vi "Convert_Algo_Info.vi"(0 "ERD Data Out 1":T1[](array[typedef]) {"ERD Number" format="%.0x"}, 5 "ERD Data Out 2":T1[](array[typedef]) {"ERD Number" format="%.0x"}, 11 "Error In":errorcluster) -> (4 "Algorithm Data":T2, 15 "Error Out":errorcluster)   [LabVIEW 2014]
uses:
  type defs/Algorithms.ctl
  Utility/Labview GEA2 Toolkit v2.1/type defs/ERD Read Data Out.ctl
  Utility/Labview GEA2 Toolkit v2.1/library/GEA2_Toolkit.lvlib
panel:
  # "Wet Load Size"
  # "Dry Load Size"
  # "OOB"
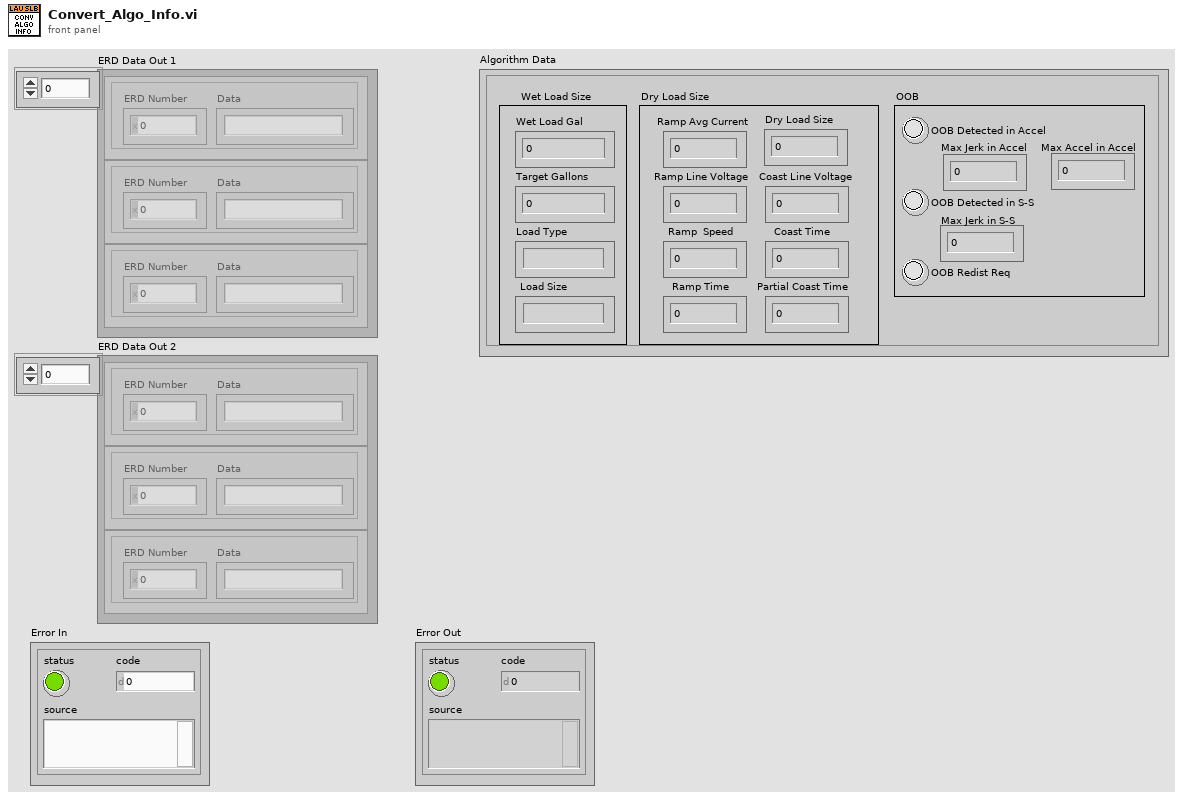
[diagram p1: front panel]
types:
  T1 = typedef "GEA2_Toolkit.lvlib/ERD Read Data Out.ctl" = cluster{"ERD Number":u16, "Data":string}
  T2 = typedef "Algorithms.ctl" = cluster{"Wet Load Gal":dbl, "Target Gallons":dbl, "Load Type":string, "Load Size":string, "Coast Time":u16, "Ramp Time":u16, "Ramp  Speed":u16, "Ramp Avg Current":dbl, "OOB Redist Req":bool, "OOB Detected in S-S":bool, "Max Accel in Accel":i32, "Max Jerk in Accel":i32, "Max Jerk in S-S":i32, "OOB Detected in Accel":bool, "Partial Coast Time":u16, "Dry Load Size":dbl, "Ramp Line Voltage ":dbl, "Coast Line Voltage":dbl}
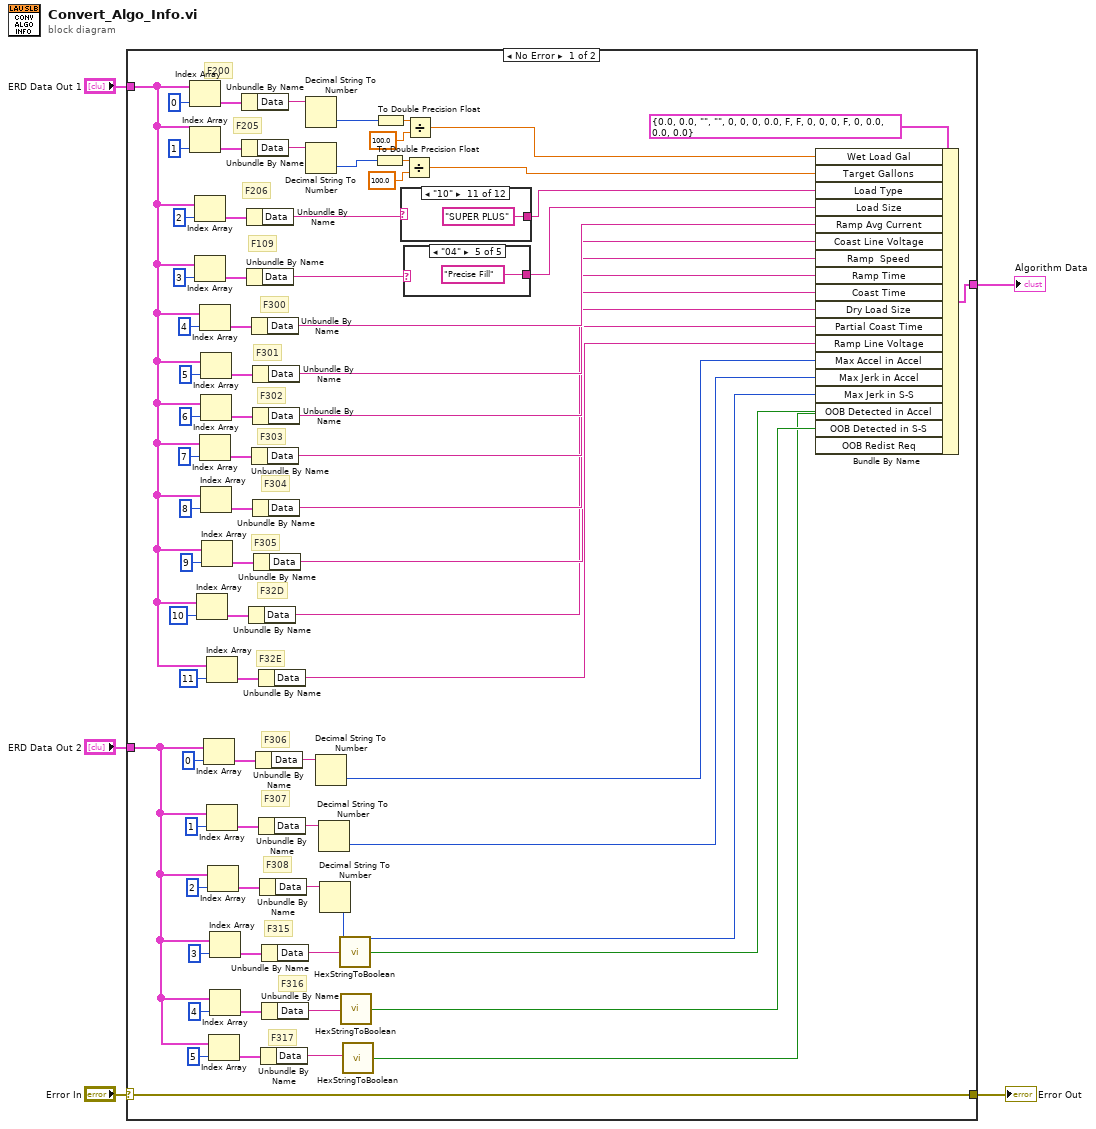
[diagram p0: block diagram]
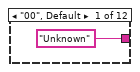
[diagram p2: hidden frame]
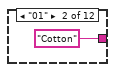
[diagram p3: hidden frame]
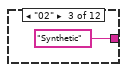
[diagram p4: hidden frame]
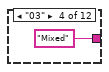
[diagram p5: hidden frame]
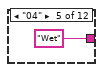
[diagram p6: hidden frame]
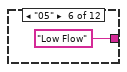
[diagram p7: hidden frame]
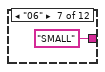
[diagram p8: hidden frame]
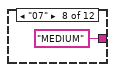
[diagram p9: hidden frame]
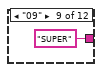
[diagram p10: hidden frame]
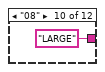
[diagram p11: hidden frame]
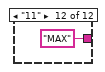
[diagram p12: hidden frame]
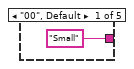
[diagram p13: hidden frame]
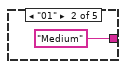
[diagram p14: hidden frame]
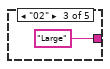
[diagram p15: hidden frame]
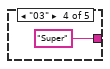
[diagram p16: hidden frame]
diagram:
  n1 = case shown="No Error" "Error In" {
    selector: "Error In" -> [w80 w98]
    tunnel: [w80 w98] -> w4
    tunnel: [w78 _] -> w3
    tunnel: "ERD Data Out 1" -> [w14 _]
    tunnel: "ERD Data Out 2" -> [w25 _]
    frame No Error {
      # "F32E"
      # "F32D"
      # "F317"
      # "F316"
      # "F315"
      # "F308"
      # "F307"
      # "F306"
      # "F305"
      # "F304"
      # "F303"
      # "F302"
      # "F301"
      # "F300"
      # "F109"
      # "F206"
      # "F205"
      # "F200"
      n2 = Index Array(array=w14, index=0) -> (element=w68:T1)
      n3 = Index Array(array=w14, index=1) -> (element=w64:T1)
      n4 = Index Array(array=w14, index=2) -> (element=w60:T1)
      n5 = Index Array(array=w14, index=3) -> (element=w56:T1)
      n6 = Index Array(array=w14, index=10) -> (element=w18:T1)
      n7 = Index Array(array=w14, index=4) -> (element=w58:T1)
      n8 = Index Array(array=w14, index=7) -> (element=w49:T1)
      n9 = Index Array(array=w14, index=5) -> (element=w53:T1)
      n10 = Index Array(array=w14, index=6) -> (element=w52:T1)
      n11 = Index Array(array=w14, index=8) -> (element=w48:T1)
      n12 = Index Array(array=w14, index=9) -> (element=w45:T1)
      n13 = Index Array(array=w25, index=0) -> (element=w44:T1)
      n14 = Index Array(array=w14, index=11) -> (element=w16:T1)
      n15 = Index Array(array=w25, index=1) -> (element=w37:T1)
      n16 = Index Array(array=w25, index=2) -> (element=w36:T1)
      n17 = Index Array(array=w25, index=5) -> (element=w26:T1)
      n18 = Index Array(array=w25, index=3) -> (element=w30:T1)
      n19 = Index Array(array=w25, index=4) -> (element=w29:T1)
      n20 = Unbundle By Name(w68) -> ("Data"=w67:string)
      n21 = Unbundle By Name(w64) -> ("Data"=w65:string)
      n22 = Unbundle By Name(w60) -> ("Data"=w59:string)
      n23 = Unbundle By Name(w56) -> ("Data"=w40:string)
      n24 = Unbundle By Name(w18) -> ("Data"=w7:string)
      n25 = Unbundle By Name(w58) -> ("Data"=w13:string)
      n26 = Unbundle By Name(w49) -> ("Data"=w10:string)
      n27 = Unbundle By Name(w53) -> ("Data"=w12:string)
      n28 = Unbundle By Name(w52) -> ("Data"=w11:string)
      n29 = Unbundle By Name(w48) -> ("Data"=w9:string)
      n30 = Unbundle By Name(w45) -> ("Data"=w8:string)
      n31 = Unbundle By Name(w44) -> ("Data"=w42:string)
      n32 = Unbundle By Name(w16) -> ("Data"=w6:string)
      n33 = Unbundle By Name(w37) -> ("Data"=w39:string)
      n34 = Unbundle By Name(w36) -> ("Data"=w34:string)
      n35 = Unbundle By Name(w26) -> ("Data"=w22:string)
      n36 = Unbundle By Name(w30) -> ("Data"=w24:string)
      n37 = Unbundle By Name(w29) -> ("Data"=w23:string)
      n38 = Decimal String To Number(string=w67) -> (number=w66:i32)  [unwired: 2 in, 1 out]
      n39 = Decimal String To Number(string=w65) -> (number=w62:i32)  [unwired: 2 in, 1 out]
      n40 = Decimal String To Number(string=w42) -> (number=w41:i32)  [unwired: 2 in, 1 out]
      n41 = Decimal String To Number(string=w39) -> (number=w33:i32)  [unwired: 2 in, 1 out]
      n42 = Decimal String To Number(string=w34) -> (number=w32:i32)  [unwired: 2 in, 1 out]
      n43 = call "HexStringToBoolean.vi"("Hex String"=w24) -> ("Boolean"=w21:bool)
      n44 = call "HexStringToBoolean.vi"("Hex String"=w23) -> ("Boolean"=w20:bool)
      n45 = call "HexStringToBoolean.vi"("Hex String"=w22) -> ("Boolean"=w19:bool)
      n46 = To Double Precision Float(number=w62) -> (double precision float=w74:dbl)
      n47 = To Double Precision Float(number=w66) -> (double precision float=w76:dbl)
      n48 = case shown="\"10\"" w59 {
        tunnel: ["Unknown" ("Load Type") "Cotton" ("Load Type") "Synthetic" ("Load Type") "Mixed" ("Load Type") "Wet" ("Load Type") "Low Flow" ("Load Type") "SMALL" ("Load Type") "MEDIUM" ("Load Type") "SUPER" ("Load Type") "LARGE" ("Load Type") "SUPER PLUS" ("Load Type") "MAX" ("Load Type")] -> w71
        frame "00", Default {
        }
        frame "01" {
        }
        frame "02" {
        }
        frame "03" {
        }
        frame "04" {
        }
        frame "05" {
        }
        frame "06" {
        }
        frame "07" {
        }
        frame "09" {
        }
        frame "08" {
        }
        frame "10" {
        }
        frame "11" {
        }
      }
      n49 = Divide(x=w74, y=100.0) -> (x/y=w72:dbl)
      n50 = case shown="\"04\"" w40 {
        tunnel: ["Small" ("Low End Load Size") "Medium" ("Low End Load Size") "Large" ("Low End Load Size") "Super" ("Low End Load Size") "Precise Fill" ("Low End Load Size")] -> w70
        frame "00", Default {
        }
        frame "01" {
        }
        frame "02" {
        }
        frame "03" {
        }
        frame "04" {
        }
      }
      n51 = Divide(x=w76, y=100.0) -> (x/y=w75:dbl)
      n52 = Bundle By Name(cluster=T2 {"Wet Load Gal"=0.0, "Target Gallons"=0.0, "Load Type"="", "Load Size"="", "Coast Time"=0, "Ramp Time"=0, "Ramp  Speed"=0, "Ramp Avg Current"=0.0, "OOB Redist Req"=FALSE, "OOB Detected in S-S"=FALSE, "Max Accel in Accel"=0, "Max Jerk in Accel"=0, "Max Jerk in S-S"=0, "OOB Detected in Accel"=FALSE, "Partial Coast Time"=0, "Dry Load Size"=0.0, "Ramp Line Voltage "=0.0, "Coast Line Voltage"=0.0} ("Algorithm Data"), "Wet Load Gal"=w75, "Target Gallons"=w72, "Load Type"=w71, "Load Size"=w70, "Ramp Avg Current"=w13, "Coast Line Voltage"=w12, "Ramp  Speed"=w11, "Ramp Time"=w10, "Coast Time"=w9, "Dry Load Size"=w8, "Partial Coast Time"=w7, "Ramp Line Voltage"=w6, "Max Accel in Accel"=w41, "Max Jerk in Accel"=w33, "Max Jerk in S-S"=w32, "OOB Detected in Accel"=w21, "OOB Detected in S-S"=w20, "OOB Redist Req"=w19) -> (w78:T2)
    }
    frame Error {
    }
  }
  "Error Out" <- w4
  "Algorithm Data" <- w3
